vi "Autonomous Independent.vi"   [LabVIEW 2017] (continued)
                tunnel: [w2150] -> w2003
                tunnel: w2006 -> [w2151]
                tunnel: [w2149] -> w2002
                tunnel: w2005 -> [w2155]
                tunnel: [w2155] -> w2001
                tunnel: w2004 -> [w2154]
                tunnel: [w2154] -> w2000
                tunnel: w2003 -> [w2168]
                tunnel: w2002 -> [w2167]
                tunnel: w2001 -> [w2166]
                tunnel: w2000 -> [w2165]
                tunnel: [w2159] -> w1999
                tunnel: [w2158] -> w1998
                tunnel: [w2157] -> w1997
                tunnel: [w2156] -> w1996
                tunnel: w1999 -> [w2175]
                tunnel: [w2175] -> w1995
                tunnel: w1998 -> [w2174]
                tunnel: [w2174] -> w1994
                tunnel: w1997 -> [w2173]
                tunnel: [w2173] -> w1993
                tunnel: w1996 -> [w2172]
                tunnel: [w2172] -> w1992
                tunnel: w1995 -> [w2180]
                tunnel: w1994 -> [w2179]
                tunnel: w1993 -> [w2177]
                tunnel: w1992 -> [w2178]
                tunnel: w1987 -> [w2176]
                frame #0 {
                  n572 = global write "Robot Global Data.vi" "Raise_Mast"(FALSE ("Current State")) -> ()
                  n573 = call "PID Distance.vi"("Distance"=20.0, "Angle"=0.0, "RightEncoder"=w2053, "LeftEncoder"=w2054, "GyroDevRef"=w2055, "RobotDriveDevRef"=w2056) -> ("RightEncoder 2"=w2052:T11, "LeftEncoder 2"=w2051:T11, "GyroDevRef 2"=w2050:T8, "RobotDriveDevRef 2"=w2049:T1)  [unwired: 2 in]
                }
                frame #1 {
                  n574 = global write "Robot Global Data.vi" "Raise_Mast"(TRUE ("Current State")) -> ()
                  n575 = call "PID Distance.vi"("Distance"=225.0, "Angle"=0.0, "RightEncoder"=w2059, "LeftEncoder"=w2060, "GyroDevRef"=w2061, "RobotDriveDevRef"=w2062) -> ("RightEncoder 2"=w2063:T11, "LeftEncoder 2"=w2064:T11, "GyroDevRef 2"=w2065:T8, "RobotDriveDevRef 2"=w2066:T1)  [unwired: 2 in]
                }
                frame #2 {
                  n576 = call "PID turning.vi"("Angle"=90.0, "GyroDevRef"=w2073, "RobotDriveDevRef"=w2072) -> ("GyroDevRef 2"=w2070:T8, "RobotDriveDevRef 2"=w2071:T1)  [unwired: 7 in]
                }
                frame #3 {
                  n577 = call <vilib>:"WPI_EncoderReset.vi"("EncoderDevRef"=w2082) -> ("EncoderDevRef"=w2080:T11)  [unwired: 9 in, 1 out]
                  n578 = Wait (ms)(milliseconds to wait=u32 10) -> ()  [unwired: 1 out]
                  n579 = call <vilib>:"WPI_EncoderReset.vi"("EncoderDevRef"=w2083) -> ("EncoderDevRef"=w2081:T11)  [unwired: 9 in, 1 out]
                }
                frame #4 {
                  n580 = global read "Robot Global Data.vi" "Axes"() -> (w2095:dbl[])
                  n581 = global write "Robot Global Data.vi" "Lift_Position"(2.0) -> ()
                  n582 = call "PID Distance.vi"("Distance"=199.0, "Angle"=90.0, "RightEncoder"=w2088, "LeftEncoder"=w2089, "GyroDevRef"=w2090, "RobotDriveDevRef"=w2091) -> ("RightEncoder 2"=w2085:T11, "LeftEncoder 2"=w2084:T11, "GyroDevRef 2"=w2087:T8, "RobotDriveDevRef 2"=w2086:T1)  [unwired: 2 in]
                  n583 = Array To Cluster(array=w2095) -> (cluster=w2094:T15)
                  n584 = Bundle By Name(cluster=w2094, "Axes[1]"=-1.0) -> (w2093:T15)
                  n585 = Cluster To Array(cluster=w2093) -> (array=w2092:dbl[])
                  n586 = global write "Robot Global Data.vi" "Axes"(w2092) -> ()
                }
                frame #5 {
                  n587 = call "PID turning.vi"("Angle"=0.0, "GyroDevRef"=w2102, "RobotDriveDevRef"=w2103) -> ("GyroDevRef 2"=w2100:T8, "RobotDriveDevRef 2"=w2101:T1)  [unwired: 7 in]
                }
                frame #6 {
                  n588 = call <vilib>:"WPI_EncoderReset.vi"("EncoderDevRef"=w2108) -> ("EncoderDevRef"=w2111:T11)  [unwired: 9 in, 1 out]
                  n589 = call <vilib>:"WPI_EncoderReset.vi"("EncoderDevRef"=w2107) -> ("EncoderDevRef"=w2110:T11)  [unwired: 9 in, 1 out]
                }
                frame #7 {
                  n590 = call "PID Distance.vi"("Distance"=38.0, "Angle"=0.0, "RightEncoder"=w2118, "LeftEncoder"=w2119, "GyroDevRef"=w2121, "RobotDriveDevRef"=w2120) -> ("RightEncoder 2"=w2114:T11, "LeftEncoder 2"=w2115:T11, "GyroDevRef 2"=w2116:T8, "RobotDriveDevRef 2"=w2117:T1)  [unwired: 2 in]
                  n591 = global write "Robot Global Data.vi" "Lift_Position"(3.0) -> ()
                }
                frame #8 {
                  n592 = call "PID turning.vi"("Angle"=-20.0, "GyroDevRef"=w2125, "RobotDriveDevRef"=w2128) -> ("GyroDevRef 2"=w2124:T8, "RobotDriveDevRef 2"=w2127:T1)  [unwired: 7 in]
                }
                frame #9 {
                  w2142 = 0.0 ("Left axis value")
                  n593 = global read "Robot Global Data.vi" "Axes"() -> (w2137:dbl[])
                  n594 = Wait (ms)(milliseconds to wait=u32 300) -> ()  [unwired: 1 out]
                  n595 = Array To Cluster(array=w2137) -> (cluster=w2136:T15)
                  n596 = Bundle By Name(cluster=w2136, "Axes[1]"=0.25) -> (w2139:T15)
                  n597 = Cluster To Array(cluster=w2139) -> (array=w2138:dbl[])
                  n598 = call <vilib>:"WPI_RobotDriveTankDrive.vi"("Right axis value"=w2142, "Left axis value"=w2142, "RobotDriveDevRef"=w2141) -> ("RobotDriveDevRef"=w2135:T1)  [unwired: 6 in, 2 out]
                  n599 = global write "Robot Global Data.vi" "Axes"(w2138) -> ()
                }
                frame #10 {
                  n600 = global write "Robot Global Data.vi" "Current State"(FALSE ("Current State")) -> ()
                  n601 = Wait (ms)(milliseconds to wait=u32 350) -> ()  [unwired: 1 out]
                }
                frame #11 {
                  n602 = call "PID turning.vi"("Angle"=0.0, "GyroDevRef"=w2151, "RobotDriveDevRef"=w2152) -> ("GyroDevRef 2"=w2149:T8, "RobotDriveDevRef 2"=w2150:T1)  [unwired: 7 in]
                }
                frame #12 {
                  n603 = global read "Robot Global Data.vi" "Axes"() -> (w2164:dbl[])
                  n604 = call "PID Distance.vi"("Distance"=20.0, "Angle"=0.0, "RightEncoder"=w2165, "LeftEncoder"=w2166, "GyroDevRef"=w2167, "RobotDriveDevRef"=w2168) -> ("RightEncoder 2"=w2156:T11, "LeftEncoder 2"=w2157:T11, "GyroDevRef 2"=w2158:T8, "RobotDriveDevRef 2"=w2159:T1)  [unwired: 2 in]
                  n605 = Array To Cluster(array=w2164) -> (cluster=w2163:T15)
                  n606 = Bundle By Name(cluster=w2163, "Axes[1]"=-1.0) -> (w2162:T15)
                  n607 = Cluster To Array(cluster=w2162) -> (array=w2161:dbl[])
                  n608 = global write "Robot Global Data.vi" "Axes"(w2161) -> ()
                }
                frame #13 {
                  n609 = global write "Robot Global Data.vi" "Lift_Position"(1.0) -> ()
                }
                frame #14 {
                  n610 = case shown="\"L\"" w2176 {
                    tunnel: w2180 -> [w2184 w2255 _]
                    tunnel: w2179 -> [w2183 w2254 _]
                    tunnel: w2178 -> [w2182 w2251 _]
                    tunnel: w2177 -> [w2181 w2250 _]
                    frame "L" {
                      n611 = flat-sequence {
                        tunnel: w2184 -> [w2193]
                        tunnel: w2183 -> [w2192]
                        tunnel: [w2195] -> w2190
                        tunnel: [w2194] -> w2189
                        tunnel: w2190 -> [w2202]
                        tunnel: w2189 -> [w2201]
                        tunnel: [w2202] -> w2185
                        tunnel: [w2201] -> w2186
                        tunnel: [w2199] -> w2187
                        tunnel: [w2198] -> w2188
                        tunnel: w2182 -> [w2197]
                        tunnel: w2181 -> [w2196]
                        tunnel: w2188 -> [w2204]
                        tunnel: w2187 -> [w2205]
                        tunnel: w2186 -> [w2206]
                        tunnel: w2185 -> [w2207]
                        frame #0 {
                          n612 = call "PID turning.vi"("Angle"=-170.0, "GyroDevRef"=w2192, "RobotDriveDevRef"=w2193) -> ("GyroDevRef 2"=w2194:T8, "RobotDriveDevRef 2"=w2195:T1)  [unwired: 7 in]
                        }
                        frame #1 {
                          n613 = call <vilib>:"WPI_EncoderReset.vi"("EncoderDevRef"=w2197) -> ("EncoderDevRef"=w2198:T11)  [unwired: 9 in, 1 out]
                          n614 = Wait (ms)(milliseconds to wait=u32 10) -> ()  [unwired: 1 out]
                          n615 = call <vilib>:"WPI_EncoderReset.vi"("EncoderDevRef"=w2196) -> ("EncoderDevRef"=w2199:T11)  [unwired: 9 in, 1 out]
                        }
                        frame #2 {
                          n616 = global read "Robot Global Data.vi" "Axes"() -> (w2213:dbl[])
                          n617 = Wait (ms)(milliseconds to wait=u32 400) -> ()  [unwired: 1 out]
                          n618 = Array To Cluster(array=w2213) -> (cluster=w2214:T15)
                          n619 = Bundle By Name(cluster=w2214, "Axes[1]"=1.0) -> (w2215:T15)
                          n620 = global read "Robot Global Data.vi" "PIXY Output"() -> (w2203:T16)
                          n621 = Unbundle By Name(w2203) -> ("SIGNATURE NUMBER"=w2210:u16)
                          n622 = global read "Robot Global Data.vi" "Cube Signature"() -> (w2208:dbl)
                          n623 = Equal?(x=w2210, y=w2208) -> (x = y?=w2209:bool)
                          n624 = Cluster To Array(cluster=w2215) -> (array=w2216:dbl[])
                          n625 = global write "Robot Global Data.vi" "Axes"(w2216) -> ()
                          n626 = case shown="False" w2209 {
                            tunnel: [w2218 w2231] -> _
                            tunnel: [w2217 w2230] -> _
                            tunnel: [w2220 w2229] -> _
                            tunnel: [w2221 w2228] -> _
                            tunnel: w2207 -> [w2219 w2225]
                            tunnel: w2206 -> [w2220 w2224]
                            tunnel: w2205 -> [w2217 w2223]
                            tunnel: w2204 -> [w2218 w2222]
                            frame True {
                              n627 = call "PID vision.vi"("RobotDriveDevRef in"=w2219) -> ("RobotDriveDevRef out"=w2221:T1)  [unwired: 9 in, 1 out]
                            }
                            frame False {
                              n628 = call "PID Distance.vi"("Distance"=45.0, "Angle"=-170.0, "RightEncoder"=w2222, "LeftEncoder"=w2223, "GyroDevRef"=w2224, "RobotDriveDevRef"=w2225) -> ("RightEncoder 2"=w2231:T11, "LeftEncoder 2"=w2230:T11, "GyroDevRef 2"=w2229:T8, "RobotDriveDevRef 2"=w2228:T1)  [unwired: 2 in]
                            }
                          }
                        }
                        frame #3 {
                          n629 = global write "Robot Global Data.vi" "Current State"(TRUE ("Current State")) -> ()
                          n630 = Wait (ms)(milliseconds to wait=u32 300) -> ()  [unwired: 1 out]
                        }
                      }
                    }
                    frame "R" {
                      n631 = flat-sequence {
                        tunnel: w2255 -> [w2258]
                        tunnel: w2254 -> [w2257]
                        tunnel: [w2260] -> w2253
                        tunnel: [w2259] -> w2252
                        tunnel: w2253 -> [w2267]
                        tunnel: w2252 -> [w2266]
                        tunnel: w2251 -> [w2264]
                        tunnel: w2250 -> [w2263]
                        tunnel: [w2267] -> w2249
                        tunnel: [w2266] -> w2248
                        tunnel: [w2262] -> w2247
                        tunnel: [w2261] -> w2246
                        tunnel: [w2285] -> w2245
                        tunnel: [w2284] -> w2244
                        tunnel: [w2283] -> w2243
                        tunnel: [w2282] -> w2242
                        tunnel: w2246 -> [w2274]
                        tunnel: w2247 -> [w2275]
                        tunnel: w2248 -> [w2273]
                        tunnel: w2249 -> [w2272]
                        tunnel: w2245 -> [w2306]
                        tunnel: w2244 -> [w2305]
                        tunnel: w2243 -> [w2304]
                        tunnel: w2242 -> [w2303]
                        tunnel: [w2306] -> w2241
                        tunnel: [w2305] -> w2239
                        tunnel: [w2304] -> w2237
                        tunnel: [w2303] -> w2235
                        tunnel: w2241 -> [w2317]
                        tunnel: [w2317] -> w2240
                        tunnel: w2239 -> [w2316]
                        tunnel: [w2316] -> w2238
                        tunnel: w2237 -> [w2315]
                        tunnel: [w2315] -> w2236
                        tunnel: w2235 -> [w2314]
                        tunnel: [w2314] -> w2234
                        tunnel: w2240 -> [w2318]
                        tunnel: w2238 -> [w2321]
                        tunnel: w2236 -> [w2320]
                        tunnel: w2234 -> [w2319]
                        frame #0 {
                          n632 = call "PID turning.vi"("Angle"=-170.0, "GyroDevRef"=w2257, "RobotDriveDevRef"=w2258) -> ("GyroDevRef 2"=w2259:T8, "RobotDriveDevRef 2"=w2260:T1)  [unwired: 7 in]
                        }
                        frame #1 {
                          n633 = call <vilib>:"WPI_EncoderReset.vi"("EncoderDevRef"=w2263) -> ("EncoderDevRef"=w2261:T11)  [unwired: 9 in, 1 out]
                          n634 = Wait (ms)(milliseconds to wait=u32 10) -> ()  [unwired: 1 out]
                          n635 = call <vilib>:"WPI_EncoderReset.vi"("EncoderDevRef"=w2264) -> ("EncoderDevRef"=w2262:T11)  [unwired: 9 in, 1 out]
                        }
                        frame #2 {
                          n636 = global read "Robot Global Data.vi" "Axes"() -> (w2278:dbl[])
                          n637 = Wait (ms)(milliseconds to wait=u32 250) -> ()  [unwired: 1 out]
                          n638 = Array To Cluster(array=w2278) -> (cluster=w2279:T15)
                          n639 = Bundle By Name(cluster=w2279, "Axes[1]"=1.0) -> (w2280:T15)
                          n640 = global read "Robot Global Data.vi" "PIXY Output"() -> (w2268:T16)
                          n641 = Unbundle By Name(w2268) -> ("SIGNATURE NUMBER"=w2271:u16)
                          n642 = global read "Robot Global Data.vi" "Cube Signature"() -> (w2269:dbl)
                          n643 = Equal?(x=w2271, y=w2269) -> (x = y?=w2270:bool)
                          n644 = Cluster To Array(cluster=w2280) -> (array=w2281:dbl[])
                          n645 = global write "Robot Global Data.vi" "Axes"(w2281) -> ()
                          n646 = case shown="False" w2270 {
                            tunnel: [w2287 w2300] -> w2285
                            tunnel: [w2286 w2299] -> w2284
                            tunnel: [w2288 w2298] -> w2283
                            tunnel: [w2289 w2297] -> w2282
                            tunnel: w2275 -> [w2286 w2294]
                            tunnel: w2274 -> [w2287 w2293]
                            tunnel: w2273 -> [w2288 w2292]
                            tunnel: w2272 -> [w2290 w2291]
                            frame True {
                              (unwired) 10.0 ("Distance")
                              n647 = call "PID vision.vi"("RobotDriveDevRef in"=w2290) -> ("RobotDriveDevRef out"=w2289:T1)  [unwired: 9 in, 1 out]
                            }
                            frame False {
                              n648 = call "PID Distance.vi"("Distance"=45.0, "Angle"=-170.0, "RightEncoder"=w2294, "LeftEncoder"=w2293, "GyroDevRef"=w2292, "RobotDriveDevRef"=w2291) -> ("RightEncoder 2"=w2300:T11, "LeftEncoder 2"=w2299:T11, "GyroDevRef 2"=w2298:T8, "RobotDriveDevRef 2"=w2297:T1)  [unwired: 2 in]
                            }
                          }
                        }
                        frame #3 {
                          n649 = global write "Robot Global Data.vi" "Current State"(TRUE ("Current State")) -> ()
                          n650 = Wait (ms)(milliseconds to wait=u32 500) -> ()  [unwired: 1 out]
                        }
                        frame #4 {
                          n651 = global read "Robot Global Data.vi" "Axes"() -> (w2312:dbl[])
                          n652 = global write "Robot Global Data.vi" "Lift_Position"(2.0) -> ()
                          n653 = Wait (ms)(milliseconds to wait=u32 250) -> ()  [unwired: 1 out]
                          n654 = Array To Cluster(array=w2312) -> (cluster=w2311:T15)
                          n655 = Bundle By Name(cluster=w2311, "Axes[1]"=-1.0) -> (w2309:T15)
                          n656 = Cluster To Array(cluster=w2309) -> (array=w2308:dbl[])
                          n657 = global write "Robot Global Data.vi" "Axes"(w2308) -> ()
                        }
                        frame #5 {
                          n658 = call "PID Distance.vi"("Distance"=55.0, "Angle"=-170.0, "RightEncoder"=w2318, "LeftEncoder"=w2321, "GyroDevRef"=w2320, "RobotDriveDevRef"=w2319) -> ()  [unwired: 2 in, 4 out]
                        }
                        frame #6 {
                          n659 = global read "Robot Global Data.vi" "Axes"() -> (w2328:dbl[])
                          n660 = Array To Cluster(array=w2328) -> (cluster=w2327:T15)
                          n661 = Bundle By Name(cluster=w2327, "Axes[1]"=1.0) -> (w2325:T15)
                          n662 = Cluster To Array(cluster=w2325) -> (array=w2324:dbl[])
                          n663 = global write "Robot Global Data.vi" "Axes"(w2324) -> ()
                        }
                        frame #7 {
                          n664 = global write "Robot Global Data.vi" "Current State"(FALSE ("Current State")) -> ()
                        }
                      }
                    }
                    frame Default {
                    }
                  }
                }
              }
            }
            frame "L" {
              n665 = flat-sequence {
                tunnel: [w2398] -> w2390
                tunnel: [w2395] -> w2389
                tunnel: [w2396] -> w2388
                tunnel: [w2397] -> w2387
                tunnel: w2334 -> [w2394]
                tunnel: w2333 -> [w2393]
                tunnel: w2332 -> [w2392]
                tunnel: w2331 -> [w2391]
                tunnel: [w2405] -> w2386
                tunnel: [w2402] -> w2385
                tunnel: [w2403] -> w2384
                tunnel: [w2404] -> w2383
                tunnel: w2390 -> [w2409]
                tunnel: w2389 -> [w2406]
                tunnel: w2388 -> [w2407]
                tunnel: w2387 -> [w2408]
                tunnel: [w2416] -> w2379
                tunnel: [w2415] -> w2380
                tunnel: [w2413] -> w2381
                tunnel: [w2414] -> w2382
                tunnel: w2386 -> [w2420]
                tunnel: w2385 -> [w2417]
                tunnel: w2384 -> [w2418]
                tunnel: w2383 -> [w2419]
                tunnel: [w2428] -> w2378
                tunnel: w2382 -> [w2424]
                tunnel: w2381 -> [w2425]
                tunnel: w2380 -> [w2427]
                tunnel: w2379 -> [w2429]
                tunnel: [w2426] -> w2377
                tunnel: [w2425] -> w2376
                tunnel: [w2424] -> w2375
                tunnel: w2378 -> [w2439]
                tunnel: [w2439] -> w2374
                tunnel: w2377 -> [w2438]
                tunnel: [w2438] -> w2373
                tunnel: [w2437] -> w2372
                tunnel: [w2436] -> w2371
                tunnel: w2376 -> [w2434]
                tunnel: w2375 -> [w2433]
                tunnel: w2374 -> [w2445]
                tunnel: [w2443] -> w2370
                tunnel: w2373 -> [w2444]
                tunnel: [w2442] -> w2369
                tunnel: w2372 -> [w2447]
                tunnel: w2371 -> [w2446]
                tunnel: [w2441] -> w2368
                tunnel: [w2440] -> w2367
                tunnel: w2370 -> [w2454]
                tunnel: [w2453] -> w2366
                tunnel: [w2452] -> w2365
                tunnel: w2369 -> [w2452]
                tunnel: [w2451] -> w2364
                tunnel: w2368 -> [w2451]
                tunnel: [w2450] -> w2363
                tunnel: w2367 -> [w2450]
                tunnel: [w2465] -> w2362
                tunnel: w2366 -> [w2465]
                tunnel: [w2464] -> w2361
                tunnel: w2365 -> [w2464]
                tunnel: [w2463] -> w2360
                tunnel: w2364 -> [w2463]
                tunnel: [w2462] -> w2359
                tunnel: w2363 -> [w2462]
                tunnel: w2362 -> [w2470]
                tunnel: w2361 -> [w2471]
                tunnel: [w2471] -> w2358
                tunnel: [w2470] -> w2357
                tunnel: [w2469] -> w2356
                tunnel: w2360 -> [w2469]
                tunnel: [w2468] -> w2355
                tunnel: w2359 -> [w2468]
                tunnel: [w2484] -> w2354
                tunnel: w2358 -> [w2486]
                tunnel: w2357 -> [w2485]
                tunnel: w2356 -> [w2481]
                tunnel: w2355 -> [w2480]
                tunnel: [w2479] -> w2353
                tunnel: [w2478] -> w2352
                tunnel: [w2477] -> w2351
                tunnel: w2354 -> [w2493]
                tunnel: w2353 -> [w2492]
                tunnel: [w2491] -> w2350
                tunnel: w2352 -> [w2491]
                tunnel: [w2490] -> w2349
                tunnel: w2351 -> [w2490]
                tunnel: [w2489] -> w2348
                tunnel: [w2488] -> w2347
                tunnel: w2350 -> [w2501]
                tunnel: w2349 -> [w2500]
                tunnel: [w2498] -> w2346
                tunnel: w2348 -> [w2498]
                tunnel: [w2497] -> w2345
                tunnel: w2347 -> [w2497]
                tunnel: [w2496] -> w2344
                tunnel: [w2495] -> w2343
                tunnel: w2346 -> [w2514]
                tunnel: w2345 -> [w2513]
                tunnel: w2344 -> [w2512]
                tunnel: w2343 -> [w2511]
                tunnel: [w2510] -> w2342
                tunnel: [w2509] -> w2341
                tunnel: [w2508] -> w2340
                tunnel: [w2507] -> w2339
                tunnel: [w2520] -> w2338
                tunnel: [w2517] -> w2337
                tunnel: [w2519] -> w2336
                tunnel: [w2518] -> w2335
                tunnel: w2339 -> [w2517]
                tunnel: w2340 -> [w2518]
                tunnel: w2341 -> [w2519]
                tunnel: w2342 -> [w2520]
                tunnel: w2338 -> [w2527]
                tunnel: w2337 -> [w2526]
                tunnel: w2336 -> [w2525]
                tunnel: w2335 -> [w2524]
                tunnel: w2330 -> [w2523]
                frame #0 {
                  n666 = call "PID Distance.vi"("Distance"=20.0, "Angle"=-2.0, "RightEncoder"=w2391, "LeftEncoder"=w2392, "GyroDevRef"=w2393, "RobotDriveDevRef"=w2394) -> ("RightEncoder 2"=w2395:T11, "LeftEncoder 2"=w2396:T11, "GyroDevRef 2"=w2397:T8, "RobotDriveDevRef 2"=w2398:T1)  [unwired: 2 in]
                }
                frame #1 {
                  n667 = call "PID Distance.vi"("Distance"=100.0, "Angle"=-2.0, "RightEncoder"=w2406, "LeftEncoder"=w2407, "GyroDevRef"=w2408, "RobotDriveDevRef"=w2409) -> ("RightEncoder 2"=w2402:T11, "LeftEncoder 2"=w2403:T11, "GyroDevRef 2"=w2404:T8, "RobotDriveDevRef 2"=w2405:T1)  [unwired: 2 in]
                  n668 = global write "Robot Global Data.vi" "Raise_Mast"(TRUE ("Current State")) -> ()
                }
                frame #2 {
                  n669 = global write "Robot Global Data.vi" "Lift_Position"(2.0) -> ()
                  n670 = call "PID Distance.vi"("Distance"=300.0, "Angle"=-2.0, "RightEncoder"=w2417, "LeftEncoder"=w2418, "GyroDevRef"=w2419, "RobotDriveDevRef"=w2420) -> ("RightEncoder 2"=w2413:T11, "LeftEncoder 2"=w2414:T11, "GyroDevRef 2"=w2415:T8, "RobotDriveDevRef 2"=w2416:T1)  [unwired: 2 in]
                  n671 = global write "Robot Global Data.vi" "Raise_Mast"(TRUE ("Current State")) -> ()
                }
                frame #3 {
                  n672 = call "PID turning.vi"("Angle"=90.0, "GyroDevRef"=w2427, "RobotDriveDevRef"=w2429) -> ("GyroDevRef 2"=w2426:T8, "RobotDriveDevRef 2"=w2428:T1)  [unwired: 7 in]
                  n673 = global write "Robot Global Data.vi" "Lift_Position"(3.0) -> ()
                  n674 = global write "Robot Global Data.vi" "Raise_Mast"(TRUE ("Current State")) -> ()
                }
                frame #4 {
                  n675 = call <vilib>:"WPI_EncoderReset.vi"("EncoderDevRef"=w2433) -> ("EncoderDevRef"=w2436:T11)  [unwired: 9 in, 1 out]
                  n676 = Wait (ms)(milliseconds to wait=u32 100) -> ()  [unwired: 1 out]
                  n677 = call <vilib>:"WPI_EncoderReset.vi"("EncoderDevRef"=w2434) -> ("EncoderDevRef"=w2437:T11)  [unwired: 9 in, 1 out]
                }
                frame #5 {
                  n678 = call "PID Distance.vi"("Distance"=25.0, "Angle"=90.0, "RightEncoder"=w2447, "LeftEncoder"=w2446, "GyroDevRef"=w2444, "RobotDriveDevRef"=w2445) -> ("RightEncoder 2"=w2440:T11, "LeftEncoder 2"=w2441:T11, "GyroDevRef 2"=w2442:T8, "RobotDriveDevRef 2"=w2443:T1)  [unwired: 2 in]
                }
                frame #6 {
                  w2455 = 0.0 ("Left axis value")
                  n679 = global read "Robot Global Data.vi" "Axes"() -> (w2458:dbl[])
                  n680 = Wait (ms)(milliseconds to wait=u32 500) -> ()  [unwired: 1 out]
                  n681 = Array To Cluster(array=w2458) -> (cluster=w2457:T15)
                  n682 = Bundle By Name(cluster=w2457, "Axes[1]"=0.25) -> (w2460:T15)
                  n683 = Cluster To Array(cluster=w2460) -> (array=w2459:dbl[])
                  n684 = call <vilib>:"WPI_RobotDriveTankDrive.vi"("Right axis value"=w2455, "Left axis value"=w2455, "RobotDriveDevRef"=w2454) -> ("RobotDriveDevRef"=w2453:T1)  [unwired: 6 in, 2 out]
                  n685 = global write "Robot Global Data.vi" "Axes"(w2459) -> ()
                }
                frame #7 {
                  n686 = global write "Robot Global Data.vi" "Current State"(FALSE ("Current State")) -> ()
                  n687 = Wait (ms)(milliseconds to wait=u32 400) -> ()  [unwired: 1 out]
                }
                frame #8 {
                  n688 = global read "Robot Global Data.vi" "Axes"() -> (w2473:dbl[])
                  n689 = Array To Cluster(array=w2473) -> (cluster=w2472:T15)
                  n690 = Bundle By Name(cluster=w2472, "Axes[1]"=-1.0) -> (w2475:T15)
                  n691 = Cluster To Array(cluster=w2475) -> (array=w2474:dbl[])
                  n692 = global write "Robot Global Data.vi" "Axes"(w2474) -> ()
                }
                frame #9 {
                  n693 = call "PID Distance.vi"("Distance"=0.0, "Angle"=90.0, "RightEncoder"=w2480, "LeftEncoder"=w2481, "GyroDevRef"=w2486, "RobotDriveDevRef"=w2485) -> ("RightEncoder 2"=w2477:T11, "LeftEncoder 2"=w2478:T11, "GyroDevRef 2"=w2479:T8, "RobotDriveDevRef 2"=w2484:T1)  [unwired: 2 in]
                }
                frame #10 {
                  n694 = global write "Robot Global Data.vi" "Lift_Position"(1.0) -> ()
                  n695 = call "PID turning.vi"("Angle"=150.0, "GyroDevRef"=w2492, "RobotDriveDevRef"=w2493) -> ("GyroDevRef 2"=w2488:T8, "RobotDriveDevRef 2"=w2489:T1)  [unwired: 7 in]
                }
                frame #11 {
                  n696 = call <vilib>:"WPI_EncoderReset.vi"("EncoderDevRef"=w2501) -> ("EncoderDevRef"=w2496:T11)  [unwired: 9 in, 1 out]
                  n697 = Wait (ms)(milliseconds to wait=u32 10) -> ()  [unwired: 1 out]
                  n698 = call <vilib>:"WPI_EncoderReset.vi"("EncoderDevRef"=w2500) -> ("EncoderDevRef"=w2495:T11)  [unwired: 9 in, 1 out]
                }
                frame #12 {
                  n699 = global read "Robot Global Data.vi" "Axes"() -> (w2504:dbl[])
                  n700 = call "PID Distance.vi"("Distance"=130.0, "Angle"=150.0, "RightEncoder"=w2511, "LeftEncoder"=w2512, "GyroDevRef"=w2513, "RobotDriveDevRef"=w2514) -> ("RightEncoder 2"=w2507:T11, "LeftEncoder 2"=w2508:T11, "GyroDevRef 2"=w2509:T8, "RobotDriveDevRef 2"=w2510:T1)  [unwired: 2 in]
                  n701 = Array To Cluster(array=w2504) -> (cluster=w2503:T15)
                  n702 = Bundle By Name(cluster=w2503, "Axes[1]"=1.0) -> (w2506:T15)
                  n703 = Cluster To Array(cluster=w2506) -> (array=w2505:dbl[])
                  n704 = global write "Robot Global Data.vi" "Axes"(w2505) -> ()
                }
                frame #13 {
                  n705 = global write "Robot Global Data.vi" "Current State"(TRUE ("Current State")) -> ()
                  n706 = Wait (ms)(milliseconds to wait=u32 500) -> ()  [unwired: 1 out]
                }
                frame #14 {
                  n707 = case shown="\"R\"" w2523 {
                    tunnel: w2527 -> [w2531 w2555 _]
                    tunnel: w2526 -> [w2530 w2552 _]
                    tunnel: w2525 -> [w2529 w2554 _]
                    tunnel: w2524 -> [w2528 w2553 _]
                    frame "L" {
                      n708 = flat-sequence {
                        tunnel: w2531 -> [w2541]
                        tunnel: w2530 -> [w2542]
                        tunnel: w2529 -> [w2540]
                        tunnel: w2528 -> [w2539]
                        frame #0 {
                          n709 = global read "Robot Global Data.vi" "Axes"() -> (w2536:dbl[])
                          n710 = global write "Robot Global Data.vi" "Lift_Position"(2.0) -> ()
                          n711 = Wait (ms)(milliseconds to wait=u32 250) -> ()  [unwired: 1 out]
                          n712 = Array To Cluster(array=w2536) -> (cluster=w2535:T15)
                          n713 = Bundle By Name(cluster=w2535, "Axes[1]"=-1.0) -> (w2538:T15)
                          n714 = Cluster To Array(cluster=w2538) -> (array=w2537:dbl[])
                          n715 = global write "Robot Global Data.vi" "Axes"(w2537) -> ()
                        }
                        frame #1 {
                          n716 = call "PID Distance.vi"("Distance"=150.0, "Angle"=170.0, "RightEncoder"=w2542, "LeftEncoder"=w2539, "GyroDevRef"=w2540, "RobotDriveDevRef"=w2541) -> ()  [unwired: 2 in, 4 out]
                        }
                        frame #2 {
                          n717 = global read "Robot Global Data.vi" "Axes"() -> (w2548:dbl[])
                          n718 = Wait (ms)(milliseconds to wait=u32 250) -> ()  [unwired: 1 out]
                          n719 = Array To Cluster(array=w2548) -> (cluster=w2547:T15)
                          n720 = Bundle By Name(cluster=w2547, "Axes[1]"=1.0) -> (w2550:T15)
                          n721 = Cluster To Array(cluster=w2550) -> (array=w2549:dbl[])
                          n722 = global write "Robot Global Data.vi" "Axes"(w2549) -> ()
                        }
                        frame #3 {
                          n723 = global write "Robot Global Data.vi" "Current State"(FALSE ("Current State")) -> ()
                        }
                      }
                    }
                    frame "R" {
                      n724 = flat-sequence {
                        tunnel: w2555 -> [w2594]
                        tunnel: [w2591] -> _
                        tunnel: w2554 -> [w2593]
                        tunnel: w2553 -> [w2592]
                        tunnel: [w2598] -> w2583
                        tunnel: [w2597] -> w2582
                        tunnel: [w2596] -> w2581
                        tunnel: [w2595] -> w2580
                        tunnel: w2552 -> [w2591]
                        tunnel: w2583 -> [w2607]
                        tunnel: w2582 -> [w2606]
                        tunnel: [w2605] -> w2579
                        tunnel: w2581 -> [w2605]
                        tunnel: [w2604] -> w2578
                        tunnel: w2580 -> [w2604]
                        tunnel: [w2603] -> w2577
                        tunnel: [w2602] -> w2576
                        tunnel: w2579 -> [w2614]
                        tunnel: w2578 -> [w2613]
                        tunnel: [w2612] -> w2575
                        tunnel: w2577 -> [w2612]
                        tunnel: [w2611] -> w2574
                        tunnel: w2576 -> [w2611]
                        tunnel: [w2610] -> w2573
                        tunnel: [w2609] -> w2572
                        tunnel: w2575 -> [w2624]
                        tunnel: w2574 -> [w2623]
                        tunnel: w2573 -> [w2622]
                        tunnel: w2572 -> [w2621]
                        tunnel: [w2620] -> w2568
                        tunnel: [w2619] -> w2569
                        tunnel: [w2617] -> w2570
                        tunnel: [w2616] -> w2571
                        tunnel: [w2630] -> w2567
                        tunnel: [w2629] -> w2566
                        tunnel: [w2628] -> w2565
                        tunnel: [w2627] -> w2564
                        tunnel: w2571 -> [w2627]
                        tunnel: w2570 -> [w2628]
                        tunnel: w2569 -> [w2629]
                        tunnel: w2568 -> [w2630]
                        tunnel: [w2640] -> w2560
                        tunnel: w2567 -> [w2640]
                        tunnel: [w2639] -> w2561
                        tunnel: w2566 -> [w2639]
                        tunnel: [w2638] -> w2562
                        tunnel: w2565 -> [w2638]
                        tunnel: [w2637] -> w2563
                        tunnel: w2564 -> [w2637]
                        tunnel: w2563 -> [w2652]
                        tunnel: [w2652] -> w2559
                        tunnel: w2562 -> [w2651]
                        tunnel: [w2651] -> w2558
                        tunnel: w2561 -> [w2650]
                        tunnel: [w2650] -> w2557
                        tunnel: w2560 -> [w2649]
                        tunnel: [w2649] -> w2556
                        tunnel: w2559 -> [w2653]
                        tunnel: w2558 -> [w2654]
                        tunnel: w2557 -> [w2655]
                        tunnel: w2556 -> [w2656]
                        frame #0 {
                          n725 = global read "Robot Global Data.vi" "Axes"() -> (w2588:dbl[])
                          n726 = global write "Robot Global Data.vi" "Lift_Position"(2.0) -> ()
                          n727 = Wait (ms)(milliseconds to wait=u32 250) -> ()  [unwired: 1 out]
                          n728 = Array To Cluster(array=w2588) -> (cluster=w2587:T15)
                          n729 = Bundle By Name(cluster=w2587, "Axes[1]"=-1.0) -> (w2590:T15)
                          n730 = Cluster To Array(cluster=w2590) -> (array=w2589:dbl[])
                          n731 = global write "Robot Global Data.vi" "Axes"(w2589) -> ()
                        }
                        frame #1 {
                          n732 = call "PID Distance.vi"("Distance"=-10.0, "Angle"=150.0, "RightEncoder"=w2591, "LeftEncoder"=w2592, "GyroDevRef"=w2593, "RobotDriveDevRef"=w2594) -> ("RightEncoder 2"=w2595:T11, "LeftEncoder 2"=w2596:T11, "GyroDevRef 2"=w2597:T8, "RobotDriveDevRef 2"=w2598:T1)  [unwired: 2 in]
                        }
                        frame #2 {
                          n733 = global write "Robot Global Data.vi" "Lift_Position"(3.0) -> ()
                          n734 = call "PID turning.vi"("Angle"=90.0, "GyroDevRef"=w2606, "RobotDriveDevRef"=w2607) -> ("GyroDevRef 2"=w2602:T8, "RobotDriveDevRef 2"=w2603:T1)  [unwired: 7 in]
                        }
                        frame #3 {
                          n735 = call <vilib>:"WPI_EncoderReset.vi"("EncoderDevRef"=w2614) -> ("EncoderDevRef"=w2610:T11)  [unwired: 9 in, 1 out]
                          n736 = Wait (ms)(milliseconds to wait=u32 10) -> ()  [unwired: 1 out]
                          n737 = call <vilib>:"WPI_EncoderReset.vi"("EncoderDevRef"=w2613) -> ("EncoderDevRef"=w2609:T11)  [unwired: 9 in, 1 out]
                        }
                        frame #4 {
                          n738 = call "PID Distance.vi"("Distance"=30.0, "Angle"=90.0, "RightEncoder"=w2621, "LeftEncoder"=w2622, "GyroDevRef"=w2623, "RobotDriveDevRef"=w2624) -> ("RightEncoder 2"=w2616:T11, "LeftEncoder 2"=w2617:T11, "GyroDevRef 2"=w2619:T8, "RobotDriveDevRef 2"=w2620:T1)  [unwired: 2 in]
                          n739 = global write "Robot Global Data.vi" "Lift_Position"(3.0) -> ()
                        }
                        frame #5 {
                          n740 = global read "Robot Global Data.vi" "Axes"() -> (w2634:dbl[])
                          n741 = Wait (ms)(milliseconds to wait=u32 500) -> ()  [unwired: 1 out]
                          n742 = Array To Cluster(array=w2634) -> (cluster=w2633:T15)
                          n743 = Bundle By Name(cluster=w2633, "Axes[1]"=0.3) -> (w2636:T15)
                          n744 = Cluster To Array(cluster=w2636) -> (array=w2635:dbl[])
                          n745 = global write "Robot Global Data.vi" "Axes"(w2635) -> ()
                        }
                        frame #6 {
                          n746 = global write "Robot Global Data.vi" "Current State"(FALSE ("Current State")) -> ()
                          n747 = Wait (ms)(milliseconds to wait=u32 400) -> ()  [unwired: 1 out]
                        }
                        frame #7 {
                          n748 = global read "Robot Global Data.vi" "Axes"() -> (w2646:dbl[])
                          n749 = Wait (ms)(milliseconds to wait=u32 250) -> ()  [unwired: 1 out]
                          n750 = Array To Cluster(array=w2646) -> (cluster=w2645:T15)
                          n751 = Bundle By Name(cluster=w2645, "Axes[1]"=-1.0) -> (w2648:T15)
                          n752 = Cluster To Array(cluster=w2648) -> (array=w2647:dbl[])
                          n753 = global write "Robot Global Data.vi" "Axes"(w2647) -> ()
                        }
                        frame #8 {
                          n754 = call "PID Distance.vi"("Distance"=0.0, "Angle"=90.0, "RightEncoder"=w2653, "LeftEncoder"=w2654, "GyroDevRef"=w2655, "RobotDriveDevRef"=w2656) -> ()  [unwired: 2 in, 4 out]
                        }
                        frame #9 {
                          n755 = global write "Robot Global Data.vi" "Lift_Position"(1.0) -> ()
                        }
                      }
                    }
                    frame Default {
                    }
                  }
                }
              }
            }
            frame Default {
              n756 = flat-sequence {
                tunnel: w2661 -> [w2669]
                tunnel: w2660 -> [w2668]
                tunnel: w2662 -> [w2666]
                tunnel: [w2667] -> w2664
                tunnel: w2663 -> [w2665]
                tunnel: w2664 -> [w2672]
                frame #0 {
                  n757 = call "PID Distance.vi"("Distance"=90.0, "Angle"=0.0, "RightEncoder"=w2665, "LeftEncoder"=w2666, "GyroDevRef"=w2668, "RobotDriveDevRef"=w2669) -> ("RobotDriveDevRef 2"=w2667:T1)  [unwired: 2 in, 3 out]
                }
                frame #1 {
                  w2673 = 0.0
                  n758 = call <vilib>:"WPI_RobotDriveTankDrive.vi"("Right axis value"=w2673, "Left axis value"=w2673, "RobotDriveDevRef"=w2672) -> ()  [unwired: 6 in, 3 out]
                }
              }
            }
          }
        }
      }
    }
    frame "Left Scale V" {
      n759 = flat-sequence {
        tunnel: w2677 -> [w2709]
        tunnel: w2679 -> [w2707]
        tunnel: w2678 -> [w2706]
        tunnel: [w2705] -> w2684
        tunnel: [w2704] -> w2683
        tunnel: [w2703] -> w2682
        tunnel: [w2702] -> w2681
        tunnel: w2676 -> [w2695]
        tunnel: w2680 -> [w2685]
        tunnel: w2674 -> [w2711]
        tunnel: w2684 -> [w2715]
        tunnel: w2683 -> [w2714]
        tunnel: w2682 -> [w2713]
        tunnel: w2681 -> [w2712]
        tunnel: w2675 -> [w2710]
        frame #0 {
          w2708 = 0.0 ("Left axis value")
          n760 = global read "Robot Global Data.vi" "Axes"() -> (w2688:dbl[])
          n761 = Multiply(x=w2695, y=1000.0) -> (x*y=w2696:dbl)
          n762 = global write "Robot Global Data.vi" "Lift_Position"(0.0) -> ()
          n763 = global write "Robot Global Data.vi" "Raise_Mast"(FALSE ("Current State")) -> ()
          n764 = global write "Robot Global Data.vi" "Current State"(TRUE ("Current State")) -> ()
          n765 = Wait (ms)(milliseconds to wait=u32 100) -> ()  [unwired: 1 out]
          n766 = Array To Cluster(array=w2688) -> (cluster=w2687:T15)
          n767 = Bundle By Name(cluster=w2687, "Axes[1]"=-1.0) -> (w2690:T15)
          n768 = Greater?(x=w2696, y=11000.0) -> (0:w2698:bool)
          n769 = Equal?(x=w2696, y=0.0) -> (x = y?=w2699:bool)
          n770 = Or(x=w2698, y=w2699) -> ()  [unwired: 1 out]
          n771 = Cluster To Array(cluster=w2690) -> (array=w2689:dbl[])
          n772 = call <vilib>:"WPI_GyroReset.vi"("GyroDevRef"=w2706) -> ("GyroDevRef"=w2702:T8)  [unwired: 9 in, 1 out]
          n773 = call <vilib>:"WPI_EncoderReset.vi"("EncoderDevRef"=w2685) -> ("EncoderDevRef"=w2704:T11)  [unwired: 9 in, 1 out]
          n774 = global write "Robot Global Data.vi" "Axes"(w2689) -> ()
          n775 = call <vilib>:"WPI_EncoderReset.vi"("EncoderDevRef"=w2707) -> ("EncoderDevRef"=w2703:T11)  [unwired: 9 in, 1 out]
          n776 = call <vilib>:"WPI_RobotDriveTankDrive.vi"("Right axis value"=w2708, "Left axis value"=w2708, "RobotDriveDevRef"=w2709) -> ("RobotDriveDevRef"=w2705:T1)  [unwired: 6 in, 2 out]
        }
        frame #1 {
          n777 = case shown="\"R\"" w2711 {
            tunnel: w2715 -> [w2717 w3074 w3410]
            tunnel: w2714 -> [w2720 w3071 w3412]
            tunnel: w2713 -> [w2719 w3072 w3411]
            tunnel: w2712 -> [w2718 w3073 w3409]
            tunnel: w2710 -> [w2716 w3070 _]
            frame "R" {
              n778 = flat-sequence {
                tunnel: [w2780] -> w2772
                tunnel: [w2779] -> w2771
                tunnel: [w2777] -> w2770
                tunnel: [w2778] -> w2769
                tunnel: w2720 -> [w2773]
                tunnel: w2719 -> [w2774]
                tunnel: w2718 -> [w2775]
                tunnel: w2717 -> [w2776]
                tunnel: w2772 -> [w2791]
                tunnel: w2771 -> [w2792]
                tunnel: [w2795] -> w2768
                tunnel: w2770 -> [w2795]
                tunnel: [w2794] -> w2767
                tunnel: w2769 -> [w2794]
                tunnel: [w2789] -> w2766
                tunnel: [w2790] -> w2765
                tunnel: w2768 -> [w2802]
                tunnel: w2767 -> [w2801]
                tunnel: [w2800] -> w2764
                tunnel: [w2799] -> w2763
                tunnel: [w2798] -> w2762
                tunnel: w2766 -> [w2798]
                tunnel: [w2796] -> w2761
                tunnel: w2765 -> [w2796]
                tunnel: w2764 -> [w2807]
                tunnel: w2763 -> [w2808]
                tunnel: w2762 -> [w2809]
                tunnel: [w2805] -> w2760
                tunnel: [w2806] -> w2759
                tunnel: w2761 -> [w2810]
                tunnel: [w2803] -> w2758
                tunnel: [w2804] -> w2757
                tunnel: w2760 -> [w2822]
                tunnel: w2759 -> [w2821]
                tunnel: [w2820] -> w2756
                tunnel: [w2819] -> w2755
                tunnel: [w2825] -> w2754
                tunnel: w2758 -> [w2825]
                tunnel: [w2824] -> w2753
                tunnel: w2757 -> [w2824]
                tunnel: w2756 -> [w2831]
                tunnel: [w2831] -> w2752
                tunnel: [w2830] -> w2751
                tunnel: [w2829] -> w2750
                tunnel: [w2828] -> w2749
                tunnel: w2755 -> [w2828]
                tunnel: w2754 -> [w2827]
                tunnel: w2753 -> [w2826]
                tunnel: w2752 -> [w2839]
                tunnel: [w2836] -> w2748
                tunnel: w2751 -> [w2838]
                tunnel: w2750 -> [w2837]
                tunnel: w2749 -> [w2840]
                tunnel: [w2835] -> w2747
                tunnel: [w2834] -> w2746
                tunnel: [w2833] -> w2745
                tunnel: w2748 -> [w2847]
                tunnel: [w2846] -> w2744
                tunnel: w2747 -> [w2844]
                tunnel: [w2843] -> w2743
                tunnel: w2746 -> [w2849]
                tunnel: [w2849] -> w2742
                tunnel: w2745 -> [w2848]
                tunnel: [w2848] -> w2741
                tunnel: w2744 -> [w2860]
                tunnel: [w2854] -> w2740
                tunnel: [w2853] -> w2739
                tunnel: w2743 -> [w2853]
                tunnel: [w2852] -> w2738
                tunnel: w2742 -> [w2852]
                tunnel: [w2851] -> w2737
                tunnel: w2741 -> [w2851]
                tunnel: w2740 -> [w2867]
                tunnel: [w2867] -> w2736
                tunnel: w2739 -> [w2866]
                tunnel: [w2866] -> w2735
                tunnel: w2738 -> [w2865]
                tunnel: [w2865] -> w2734
                tunnel: w2737 -> [w2864]
                tunnel: [w2864] -> w2733
                tunnel: w2736 -> [w2871]
                tunnel: [w2869] -> w2732
                tunnel: w2735 -> [w2870]
                tunnel: [w2868] -> w2731
                tunnel: w2734 -> [w2874]
                tunnel: [w2874] -> w2730
                tunnel: w2733 -> [w2873]
                tunnel: [w2873] -> w2729
                tunnel: w2732 -> [w2887]
                tunnel: w2731 -> [w2886]
                tunnel: w2730 -> [w2885]
                tunnel: w2729 -> [w2884]
                tunnel: [w2878] -> w2728
                tunnel: [w2877] -> w2727
                tunnel: [w2876] -> w2726
                tunnel: [w2875] -> w2725
                tunnel: w2728 -> [w2894]
                tunnel: [w2894] -> w2724
                tunnel: w2727 -> [w2893]
                tunnel: [w2893] -> w2723
                tunnel: w2726 -> [w2892]
                tunnel: [w2892] -> w2722
                tunnel: w2725 -> [w2891]
                tunnel: [w2891] -> w2721
                tunnel: w2724 -> [w2899]
                tunnel: w2723 -> [w2898]
                tunnel: w2722 -> [w2896]
                tunnel: w2721 -> [w2897]
                tunnel: w2716 -> [w2895]
                frame #0 {
                  n779 = while {
                    stop <- w2783 stop-if-true
                    w2784 = 20.0 ("y")
                    n780 = global read "Robot Global Data.vi" "Distance 2"() -> (w2785:dbl)
                    n781 = global read "Robot Global Data.vi" "Distance"() -> (w2786:dbl)
                    n782 = Greater?(x=w2786, y=w2784) -> (0:w2788:bool)
                    n783 = Greater?(x=w2785, y=w2784) -> (0:w2787:bool)
                    n784 = And(x=w2788, y=w2787) -> (x .and. y?=w2783:bool)
                    n785 = global write "Robot Global Data.vi" "Raise_Mast"(w2783) -> ()
                  }
                  n786 = call "PID Distance.vi"("Distance"=225.0, "Angle"=0.0, "RightEncoder"=w2773, "LeftEncoder"=w2774, "GyroDevRef"=w2775, "RobotDriveDevRef"=w2776) -> ("RightEncoder 2"=w2777:T11, "LeftEncoder 2"=w2778:T11, "GyroDevRef 2"=w2779:T8, "RobotDriveDevRef 2"=w2780:T1)  [unwired: 2 in]
                }
                frame #1 {
                  n787 = call "PID turning.vi"("Angle"=90.0, "GyroDevRef"=w2792, "RobotDriveDevRef"=w2791) -> ("GyroDevRef 2"=w2789:T8, "RobotDriveDevRef 2"=w2790:T1)  [unwired: 7 in]
                }
                frame #2 {
                  n788 = call <vilib>:"WPI_EncoderReset.vi"("EncoderDevRef"=w2801) -> ("EncoderDevRef"=w2799:T11)  [unwired: 9 in, 1 out]
                  n789 = Wait (ms)(milliseconds to wait=u32 10) -> ()  [unwired: 1 out]
                  n790 = call <vilib>:"WPI_EncoderReset.vi"("EncoderDevRef"=w2802) -> ("EncoderDevRef"=w2800:T11)  [unwired: 9 in, 1 out]
                }
                frame #3 {
                  n791 = global read "Robot Global Data.vi" "Axes"() -> (w2814:dbl[])
                  n792 = call "PID Distance.vi"("Distance"=199.0, "Angle"=90.0, "RightEncoder"=w2807, "LeftEncoder"=w2808, "GyroDevRef"=w2809, "RobotDriveDevRef"=w2810) -> ("RightEncoder 2"=w2804:T11, "LeftEncoder 2"=w2803:T11, "GyroDevRef 2"=w2806:T8, "RobotDriveDevRef 2"=w2805:T1)  [unwired: 2 in]
                  n793 = global write "Robot Global Data.vi" "Lift_Position"(2.0) -> ()
                  n794 = Array To Cluster(array=w2814) -> (cluster=w2813:T15)
                  n795 = Bundle By Name(cluster=w2813, "Axes[1]"=-1.0) -> (w2812:T15)
                  n796 = Cluster To Array(cluster=w2812) -> (array=w2811:dbl[])
                  n797 = global write "Robot Global Data.vi" "Axes"(w2811) -> ()
                }
                frame #4 {
                  n798 = call "PID turning.vi"("Angle"=0.0, "GyroDevRef"=w2821, "RobotDriveDevRef"=w2822) -> ("GyroDevRef 2"=w2819:T8, "RobotDriveDevRef 2"=w2820:T1)  [unwired: 7 in]
                }
                frame #5 {
                  n799 = call <vilib>:"WPI_EncoderReset.vi"("EncoderDevRef"=w2827) -> ("EncoderDevRef"=w2830:T11)  [unwired: 9 in, 1 out]
                  n800 = call <vilib>:"WPI_EncoderReset.vi"("EncoderDevRef"=w2826) -> ("EncoderDevRef"=w2829:T11)  [unwired: 9 in, 1 out]
                }
                frame #6 {
                  n801 = call "PID Distance.vi"("Distance"=38.0, "Angle"=0.0, "RightEncoder"=w2837, "LeftEncoder"=w2838, "GyroDevRef"=w2840, "RobotDriveDevRef"=w2839) -> ("RightEncoder 2"=w2833:T11, "LeftEncoder 2"=w2834:T11, "GyroDevRef 2"=w2835:T8, "RobotDriveDevRef 2"=w2836:T1)  [unwired: 2 in]
                  n802 = global write "Robot Global Data.vi" "Lift_Position"(3.0) -> ()
                }
                frame #7 {
                  n803 = call "PID turning.vi"("Angle"=-20.0, "GyroDevRef"=w2844, "RobotDriveDevRef"=w2847) -> ("GyroDevRef 2"=w2843:T8, "RobotDriveDevRef 2"=w2846:T1)  [unwired: 7 in]
                }
                frame #8 {
                  w2861 = 0.0 ("Left axis value")
                  n804 = global read "Robot Global Data.vi" "Axes"() -> (w2856:dbl[])
                  n805 = Wait (ms)(milliseconds to wait=u32 300) -> ()  [unwired: 1 out]
                  n806 = Array To Cluster(array=w2856) -> (cluster=w2855:T15)
                  n807 = Bundle By Name(cluster=w2855, "Axes[1]"=0.25) -> (w2858:T15)
                  n808 = Cluster To Array(cluster=w2858) -> (array=w2857:dbl[])
                  n809 = call <vilib>:"WPI_RobotDriveTankDrive.vi"("Right axis value"=w2861, "Left axis value"=w2861, "RobotDriveDevRef"=w2860) -> ("RobotDriveDevRef"=w2854:T1)  [unwired: 6 in, 2 out]
                  n810 = global write "Robot Global Data.vi" "Axes"(w2857) -> ()
                }
                frame #9 {
                  n811 = global write "Robot Global Data.vi" "Current State"(FALSE ("Current State")) -> ()
                  n812 = Wait (ms)(milliseconds to wait=u32 400) -> ()  [unwired: 1 out]
                }
                frame #10 {
                  n813 = call "PID turning.vi"("Angle"=0.0, "GyroDevRef"=w2870, "RobotDriveDevRef"=w2871) -> ("GyroDevRef 2"=w2868:T8, "RobotDriveDevRef 2"=w2869:T1)  [unwired: 7 in]
                }
                frame #11 {
                  n814 = global read "Robot Global Data.vi" "Axes"() -> (w2883:dbl[])
                  n815 = Array To Cluster(array=w2883) -> (cluster=w2882:T15)
                  n816 = call "PID Distance.vi"("Distance"=0.0, "Angle"=0.0, "RightEncoder"=w2884, "LeftEncoder"=w2885, "GyroDevRef"=w2886, "RobotDriveDevRef"=w2887) -> ("RightEncoder 2"=w2875:T11, "LeftEncoder 2"=w2876:T11, "GyroDevRef 2"=w2877:T8, "RobotDriveDevRef 2"=w2878:T1)  [unwired: 2 in]
                  n817 = Bundle By Name(cluster=w2882, "Axes[1]"=-1.0) -> (w2881:T15)
                  n818 = Cluster To Array(cluster=w2881) -> (array=w2880:dbl[])
                  n819 = global write "Robot Global Data.vi" "Axes"(w2880) -> ()
                }
                frame #12 {
                  n820 = global write "Robot Global Data.vi" "Lift_Position"(1.0) -> ()
                }
                frame #13 {
                  n821 = case shown="Default" w2895 {
                    tunnel: w2899 -> [w2903 w2978 _]
                    tunnel: w2898 -> [w2902 w2977 _]
                    tunnel: w2897 -> [w2901 w2974 _]
                    tunnel: w2896 -> [w2900 w2973 _]
                    frame "L" {
                      n822 = flat-sequence {
                        tunnel: w2903 -> [w2912]
                        tunnel: w2902 -> [w2911]
                        tunnel: [w2914] -> w2909
                        tunnel: [w2913] -> w2908
                        tunnel: w2909 -> [w2921]
                        tunnel: w2908 -> [w2920]
                        tunnel: [w2921] -> w2904
                        tunnel: [w2920] -> w2905
                        tunnel: [w2918] -> w2906
                        tunnel: [w2917] -> w2907
                        tunnel: w2901 -> [w2916]
                        tunnel: w2900 -> [w2915]
                        tunnel: w2907 -> [w2923]
                        tunnel: w2906 -> [w2924]
                        tunnel: w2905 -> [w2925]
                        tunnel: w2904 -> [w2926]
                        frame #0 {
                          n823 = call "PID turning.vi"("Angle"=170.0, "GyroDevRef"=w2911, "RobotDriveDevRef"=w2912) -> ("GyroDevRef 2"=w2913:T8, "RobotDriveDevRef 2"=w2914:T1)  [unwired: 7 in]
                        }
                        frame #1 {
                          n824 = call <vilib>:"WPI_EncoderReset.vi"("EncoderDevRef"=w2915) -> ("EncoderDevRef"=w2918:T11)  [unwired: 9 in, 1 out]
                          n825 = call <vilib>:"WPI_EncoderReset.vi"("EncoderDevRef"=w2916) -> ("EncoderDevRef"=w2917:T11)  [unwired: 9 in, 1 out]
                          n826 = Wait (ms)(milliseconds to wait=u32 10) -> ()  [unwired: 1 out]
                        }
                        frame #2 {
                          n827 = global read "Robot Global Data.vi" "Axes"() -> (w2932:dbl[])
                          n828 = Wait (ms)(milliseconds to wait=u32 400) -> ()  [unwired: 1 out]
                          n829 = Array To Cluster(array=w2932) -> (cluster=w2933:T15)
                          n830 = global read "Robot Global Data.vi" "PIXY Output"() -> (w2922:T16)
                          n831 = Bundle By Name(cluster=w2933, "Axes[1]"=1.0) -> (w2934:T15)
                          n832 = Unbundle By Name(w2922) -> ("SIGNATURE NUMBER"=w2929:u16)
                          n833 = global read "Robot Global Data.vi" "Cube Signature"() -> (w2927:dbl)
                          n834 = Equal?(x=w2929, y=w2927) -> (x = y?=w2928:bool)
                          n835 = Cluster To Array(cluster=w2934) -> (array=w2935:dbl[])
                          n836 = global write "Robot Global Data.vi" "Axes"(w2935) -> ()
                          n837 = case shown="True" w2928 {
                            tunnel: [w2937 w2950] -> _
                            tunnel: [w2936 w2949] -> _
                            tunnel: [w2939 w2948] -> _
                            tunnel: [w2940 w2947] -> _
                            tunnel: w2926 -> [w2938 w2944]
                            tunnel: w2925 -> [w2939 w2943]
                            tunnel: w2924 -> [w2936 w2942]
                            tunnel: w2923 -> [w2937 w2941]
                            frame True {
                              n838 = call "PID vision.vi"("RobotDriveDevRef in"=w2938) -> ("RobotDriveDevRef out"=w2940:T1)  [unwired: 9 in, 1 out]
                            }
                            frame False {
                              n839 = call "PID Distance.vi"("Distance"=45.0, "Angle"=170.0, "RightEncoder"=w2941, "LeftEncoder"=w2942, "GyroDevRef"=w2943, "RobotDriveDevRef"=w2944) -> ("RightEncoder 2"=w2950:T11, "LeftEncoder 2"=w2949:T11, "GyroDevRef 2"=w2948:T8, "RobotDriveDevRef 2"=w2947:T1)  [unwired: 2 in]
                            }
                          }
                        }
                        frame #3 {
                          n840 = global write "Robot Global Data.vi" "Current State"(TRUE ("Current State")) -> ()
                          n841 = Wait (ms)(milliseconds to wait=u32 300) -> ()  [unwired: 1 out]
                        }
                      }
                    }
                    frame "R" {
                      n842 = flat-sequence {
                        tunnel: w2978 -> [w2981]
                        tunnel: w2977 -> [w2980]
                        tunnel: [w2983] -> w2976
                        tunnel: [w2982] -> w2975
                        tunnel: w2976 -> [w2991]
                        tunnel: w2975 -> [w2990]
                        tunnel: w2974 -> [w2988]
                        tunnel: w2973 -> [w2987]
                        tunnel: [w2991] -> w2972
                        tunnel: [w2990] -> w2971
                        tunnel: [w2986] -> w2970
                        tunnel: [w2985] -> w2969
                        tunnel: [w3009] -> w2960
                        tunnel: [w3008] -> w2958
                        tunnel: [w3007] -> w2956
                        tunnel: [w3006] -> w2954
                        tunnel: w2969 -> [w2998]
                        tunnel: w2970 -> [w2999]
                        tunnel: w2971 -> [w2997]
                        tunnel: w2972 -> [w2996]
                        tunnel: w2960 -> [w3027]
                        tunnel: [w3023] -> w2959
                        tunnel: w2958 -> [w3028]
                        tunnel: [w3024] -> w2957
                        tunnel: w2956 -> [w3029]
                        tunnel: [w3025] -> w2955
                        tunnel: w2954 -> [w3030]
                        tunnel: [w3026] -> w2953
                        tunnel: w2959 -> [w3037]
                        tunnel: w2957 -> [w3036]
                        tunnel: w2955 -> [w3035]
                        tunnel: w2953 -> [w3034]
                        tunnel: [w3037] -> w2968
                        tunnel: [w3036] -> w2966
                        tunnel: [w3035] -> w2964
                        tunnel: [w3034] -> w2962
                        tunnel: w2968 -> [w3048]
                        tunnel: [w3048] -> w2967
                        tunnel: w2966 -> [w3047]
                        tunnel: [w3047] -> w2965
                        tunnel: w2964 -> [w3046]
                        tunnel: [w3046] -> w2963
                        tunnel: w2962 -> [w3045]
                        tunnel: [w3045] -> w2961
                        tunnel: w2967 -> [w3050]
                        tunnel: w2965 -> [w3053]
                        tunnel: w2963 -> [w3052]
                        tunnel: w2961 -> [w3051]
                        frame #0 {
                          n843 = call "PID turning.vi"("Angle"=-170.0, "GyroDevRef"=w2980, "RobotDriveDevRef"=w2981) -> ("GyroDevRef 2"=w2982:T8, "RobotDriveDevRef 2"=w2983:T1)  [unwired: 7 in]
                        }
                        frame #1 {
                          n844 = call <vilib>:"WPI_EncoderReset.vi"("EncoderDevRef"=w2987) -> ("EncoderDevRef"=w2985:T11)  [unwired: 9 in, 1 out]
                          n845 = global write "Robot Global Data.vi" "Lift_Position"(0.0) -> ()
                          n846 = Wait (ms)(milliseconds to wait=u32 10) -> ()  [unwired: 1 out]
                          n847 = call <vilib>:"WPI_EncoderReset.vi"("EncoderDevRef"=w2988) -> ("EncoderDevRef"=w2986:T11)  [unwired: 9 in, 1 out]
                        }
                        frame #2 {
                          n848 = global read "Robot Global Data.vi" "Axes"() -> (w3002:dbl[])
                          n849 = Wait (ms)(milliseconds to wait=u32 400) -> ()  [unwired: 1 out]
                          n850 = Array To Cluster(array=w3002) -> (cluster=w3003:T15)
                          n851 = Bundle By Name(cluster=w3003, "Axes[1]"=1.0) -> (w3004:T15)
                          n852 = global read "Robot Global Data.vi" "PIXY Output"() -> (w2992:T16)
                          n853 = Unbundle By Name(w2992) -> ("SIGNATURE NUMBER"=w2995:u16)
                          n854 = global read "Robot Global Data.vi" "Cube Signature"() -> (w2993:dbl)
                          n855 = Equal?(x=w2995, y=w2993) -> (x = y?=w2994:bool)
                          n856 = Cluster To Array(cluster=w3004) -> (array=w3005:dbl[])
                          n857 = global write "Robot Global Data.vi" "Axes"(w3005) -> ()
                          n858 = case shown="False" w2994 {
                            tunnel: [w3013 w3017] -> w3009
                            tunnel: [w3012 w3018] -> w3008
                            tunnel: [w3011 w3019] -> w3007
                            tunnel: [w3015 w3020] -> w3006
                            tunnel: w2999 -> [w3012 w3018]
                            tunnel: w2998 -> [w3013 w3017]
                            tunnel: w2997 -> [w3014 w3019]
                            tunnel: w2996 -> [w3016 w3020]
                            frame True {
                              n859 = call <vilib>:"WPI_GyroGetAngle.vi"("GyroDevRef"=w3014) -> ("Angle"=w3010:dbl, "GyroDevRef"=w3011:T8)  [unwired: 6 in, 3 out]
                              n860 = global write "Robot Global Data.vi" "Tracked Angle"(w3010) -> ()
                              n861 = call "PID vision.vi"("RobotDriveDevRef in"=w3016) -> ("RobotDriveDevRef out"=w3015:T1)  [unwired: 9 in, 1 out]
                            }
                            frame False {
                              n862 = global write "Robot Global Data.vi" "Tracked Angle"(-170.0) -> ()
                            }
                          }
                        }
                        frame #3 {
                          n863 = global read "Robot Global Data.vi" "Tracked Angle"() -> (w3022:dbl)
